vi "Initialisation.vi"(4 "Error In":errorcluster caption="Entrée d'erreur") -> (0 "Error Out":errorcluster caption="Sortie d'erreur", 2 "ConfigurationTotale":T1, 3 "NomProjetOUT":string)   [LabVIEW 2017]
uses:
  DefDeType/ConfigTotale.ctl
  DefDeType/VoltageChannels.ctl
  DefDeType/WBridgeChannels.ctl
  DefDeType/Configuration.ctl
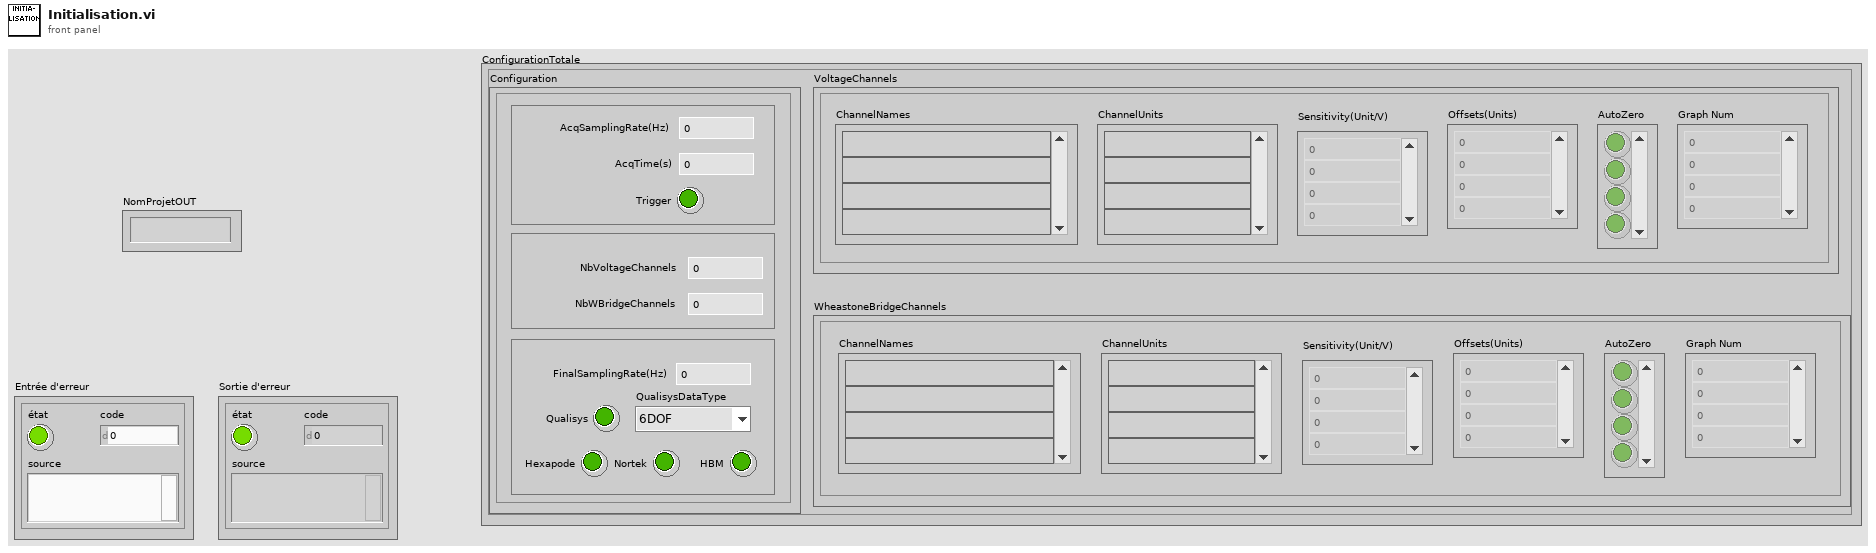
[diagram p1: front panel]
types:
  T1 = typedef "ConfigTotale.ctl" = cluster{"VoltageChannels":T2, "WheastoneBridgeChannels":T3, "Configuration":T4}
  T2 = typedef "VoltageChannels.ctl" = cluster{"ChannelNames":string[], "Sensitivity(Unit/V)":dbl[], "AutoZero":bool[], "ChannelUnits":string[], "Offsets(Units)":dbl[], "Graph Num":u8[]}
  T3 = typedef "WBridgeChannels.ctl" = cluster{"ChannelNames":string[], "Sensitivity(Unit/V)":dbl[], "AutoZero":bool[], "ChannelUnits":string[], "Offsets(Units)":dbl[], "Graph Num":u8[]}
  T4 = typedef "Configuration.ctl" = cluster{"AcqSamplingRate(Hz)":u32, "AcqTime(s)":u32, "Trigger":bool, "NbVoltageChannels":u32, "NbWBridgeChannels":u32, "Qualisys":bool, "Hexapode":bool, "FinalSamplingRate(Hz)":u32, "QualisysDataType":enum16{"6DOF", "3DTracking", "6DOF + 3D"}, "Nortek":bool, "HBM":bool}
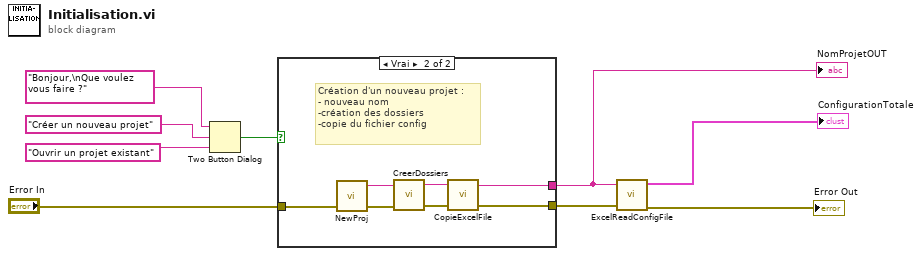
[diagram p0: block diagram]
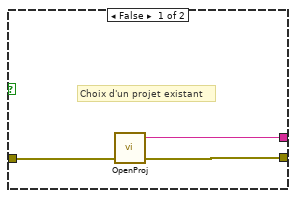
[diagram p2: hidden frame]
diagram:
  n1 = Two Button Dialog(message="Bonjour,\nQue voulez vous faire ?", 1:"Ouvrir un projet existant" ("Nom du bouton F (\"Annuler\")"), 2:"Créer un nouveau projet" ("Nom du bouton V (\"OK\")")) -> (T button?=w6:bool)
  n2 = case shown="Vrai" w6 {
    tunnel: "Error In" -> [w12 w19]
    tunnel: [w11 w15] -> w4
    tunnel: [w10 w13] -> w3
    frame False {
      # "Choix d'un projet existant"
      n3 = call "OpenProj.vi"("entrée d'erreur"=w12) -> ("sortie d'erreur"=w11:errorcluster, "NomProjet"=w10:string)  [unwired: 3 in]
    }
    frame True {
      # "Création d'un nouveau projet :\n- nouveau nom\n-création des dossiers\n-copie du fichier config"
      n4 = call "NewProj.vi"("entrée d'erreur"=w19) -> ("sortie d'erreur"=w17:errorcluster, "NomProjet"=w18:string)  [unwired: 3 in]
      n5 = call "CreerDossiers.vi"("Entrée d'erreur"=w17, "NomProjet"=w18) -> ("error out"=w16:errorcluster, "NomProjetOut"=w14:string)  [unwired: 2 in]
      n6 = call "CopieExcelFile.vi"("Entrée d'erreur"=w16, "NomProjet"=w14) -> ("sortie d'erreur"=w15:errorcluster, "NomProjetOut"=w13:string)  [unwired: 2 in]
    }
  }
  "NomProjetOUT" <- w3
  n7 = call "ExcelReadConfigFile.vi"("NomProjet"=w3, "error in (no error)"=w4) -> ("ConfigurationTotale"=→"ConfigurationTotale":T1, "error out"=→"Error Out":errorcluster)  [unwired: 3 in]
